vi "Self-Test.vi"(0 "VISA resource name":refnum<visa-resource-name>, 5 "error in (no error)":errorcluster) -> (14 "VISA resource name out":refnum<visa-resource-name>, 17 "Self-Test Error":u32, 18 "Self-Test Response":string, 19 "error out":errorcluster)   [LabVIEW 2009, in "Keithley 2000.lvlib"]
doc: "This VI causes the instrument to perform a checksum ROM test. A value of 0 indicates a successful test."
uses:
  <instrlib>/Keithley 2000/Keithley 2000.lvlib
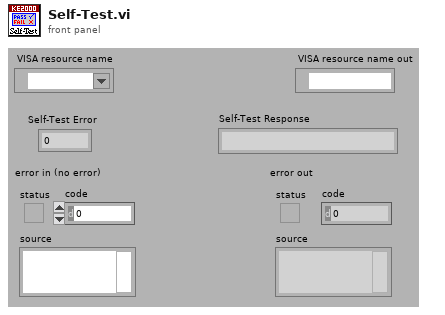
[diagram p1: front panel]
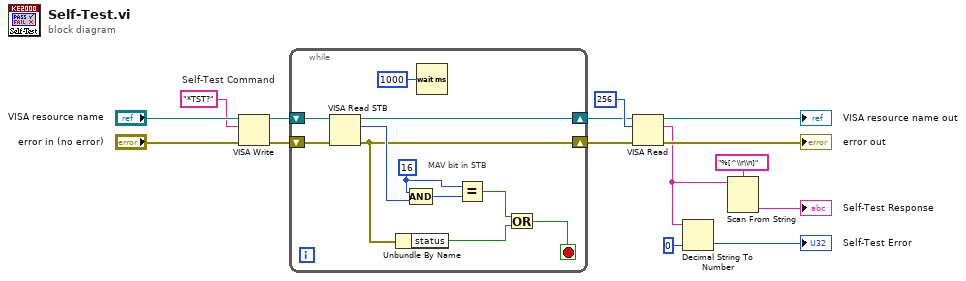
[diagram p0: block diagram]
diagram:
  w8 = "*TST?"  # Self-Test Command
  n1 = VISA Write(VISA resource name="VISA resource name", write buffer=w8, error in (no error)="error in (no error)") -> (VISA resource name out=w4:refnum<visa-resource-name>, error out=w3:errorcluster)  [unwired: 1 out]
  n2 = while {
    shift-right: [w19] -> w1
    shift-left: w3 -> [w23]
    shift-right: [w21] -> w2
    shift-left: w4 -> [w22]
    stop <- w16 stop-if-true
    w26 = u16 16 ("value")
    # "MAV bit in STB"
    n3 = VISA Read STB(8:w23, 11:w22) -> (0:w19:errorcluster, 2:w24:u16, 3:w21:refnum<visa-resource-name>)
    n4 = Unbundle By Name(w19) -> ("status"=w17:bool)
    n5 = Compound Arithmetic op=AND(w26, w24) -> (w25:u16)
    n6 = Wait (ms)(milliseconds to wait=u32 1000) -> ()  [unwired: 1 out]
    n7 = Equal?(x=w26, y=w25) -> (x = y?=w18:bool)
    n8 = Or(x=w18, y=w17) -> (x .or. y?=w16:bool)
  }
  n9 = VISA Read(VISA resource name=w2, byte count=u32 256, error in (no error)=w1) -> (VISA resource name out=→"VISA resource name out":refnum<visa-resource-name>, read buffer=w5:string, error out=→"error out":errorcluster)  [unwired: 1 out]
  n10 = Decimal String To Number(string=w5, default (0L)=u32 0 ("Default (0L)")) -> (number=→"Self-Test Error":u32)  [unwired: 1 in, 1 out]
  n11 = Scan From String(format string="%[^\\r\\n]", input string=w5) -> (output 1=→"Self-Test Response":string)  [unwired: 3 in, 3 out]
